vi "Query String.vi"(11 "URI in":refnum<class "URI.lvclass">) -> (2 "Query String":string, 3 "URI out":refnum<class "URI.lvclass">)   [LabVIEW 2020, in "URI.lvlib" / "URI.lvclass"]
uses:
  URI.lvclass
  URI.lvclass/URI.ctl
  URI.lvlib
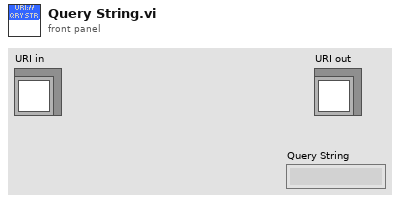
[diagram p1: front panel]
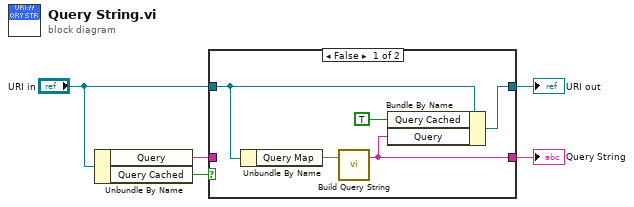
[diagram p0: block diagram]
diagram:
  n1 = Unbundle By Name("URI in") -> ("Query"=w5:string, "Query Cached"=w4:bool)
  n2 = case shown="False" w4 {
    tunnel: w5 -> [_ w12]
    tunnel: [w7 w12] -> w1
    tunnel: "URI in" -> [w10 w11]
    tunnel: [w8 w11] -> w2
    frame False {
      n3 = Unbundle By Name(w10) -> ("Query Map"=w6:map{string, string})
      n4 = call "Build Query String.vi"("Query Map"=w6) -> ("Query String"=w7:string)  [unwired: 6 in]
      n5 = Bundle By Name(cluster=w10, "Query Cached"=TRUE ("String Cached"), "Query"=w7) -> (w8:refnum<class "URI.lvclass">)
    }
    frame True {
    }
  }
  "URI out" <- w2
  "Query String" <- w1
